vi "lecroy channels to runs.vi"(8 "error in":errorcluster, 9 "Channels in Group":dbl[](array[numeric]), 10 "Crate":i32, 11 "Group Name":string) -> (0 "error out":errorcluster, 2 "Num Channels":i32[](array[numeric]), 3 "First Channel":T1[](array[typedef]) {"Card.Channel" format="%.2f"})   [LabVIEW 2018]
uses:
  archive/CAEN_SY527 v3/CAEN_SY527/subvis/channel.ctl
  <userlib>/_OpenG.lib/array/array.llb/Remove Duplicates from 1D Array (DBL)__ogtk.vi
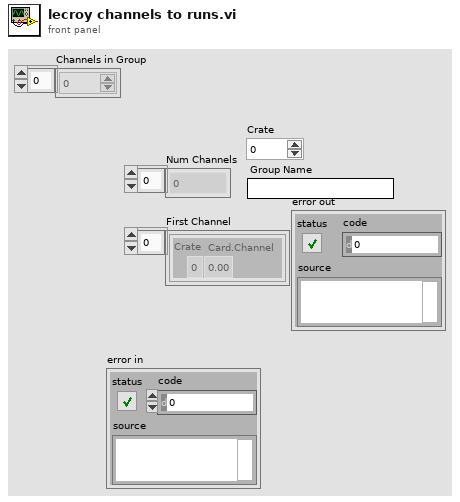
[diagram p1: front panel]
types:
  T1 = typedef "channel.ctl" = cluster{" Card.Channel":dbl, "Crate":i32}
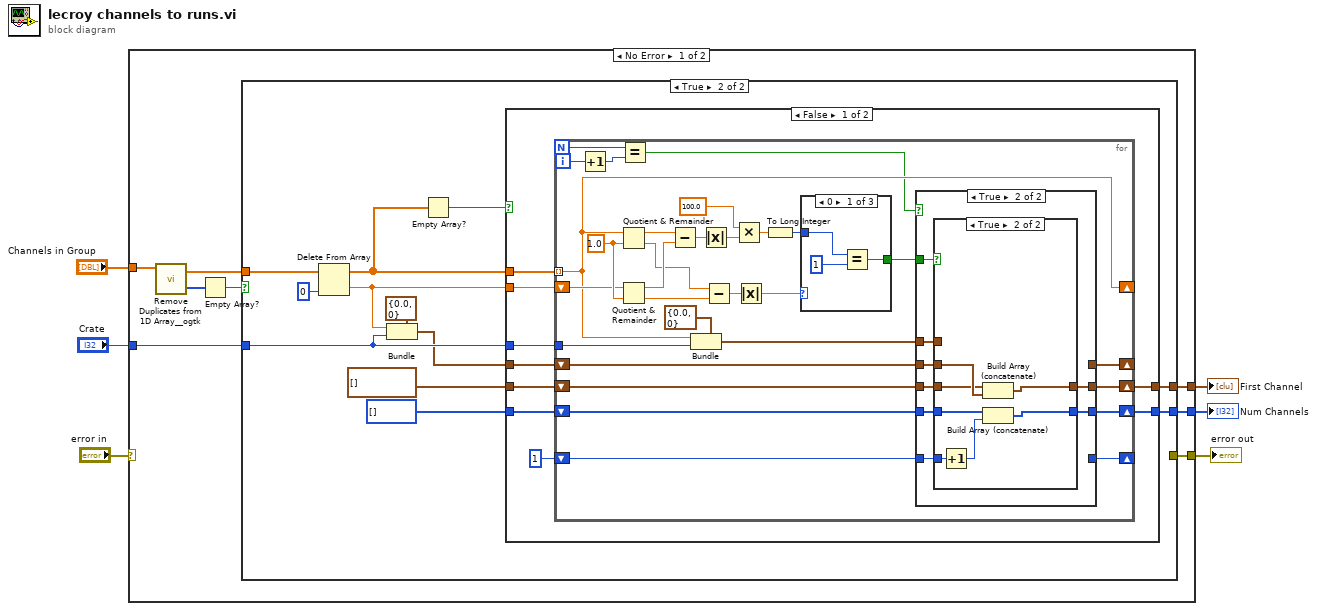
[diagram p0: block diagram]
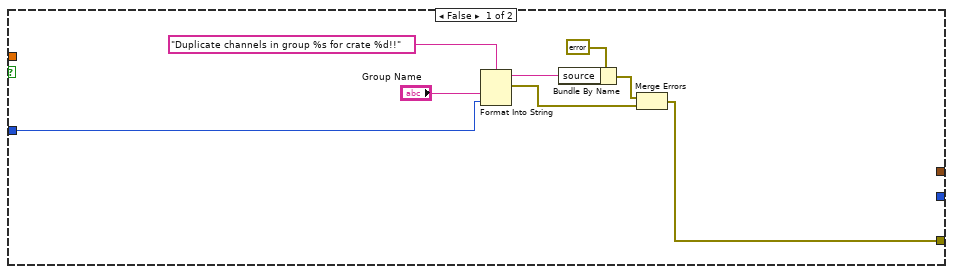
[diagram p2: hidden frame]
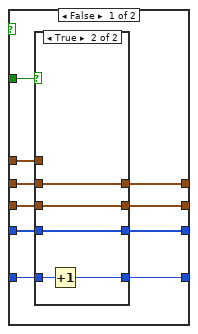
[diagram p3: hidden frame]
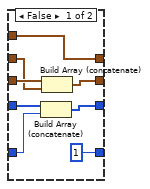
[diagram p4: hidden frame]
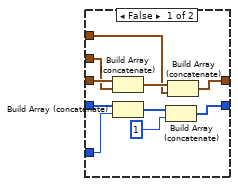
[diagram p5: hidden frame]
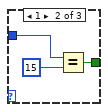
[diagram p6: hidden frame]
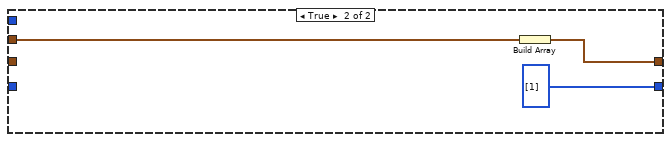
[diagram p8: hidden frame]
diagram:
  n1 = case shown="No Error" "error in" {
    selector: "error in" -> [_ w131]
    tunnel: [w14 _] -> w6
    tunnel: [w13 _] -> w5
    tunnel: "Crate" -> [w12 _]
    tunnel: "Channels in Group" -> [w11 _]
    tunnel: [w7 w131] -> w2
    frame No Error {
      n2 = call-poly <userlib>:"Remove Duplicates from 1D Array__ogtk.vi"("Input Array"=w11) -> ("Output Array"=w10:dbl[], "indices of removed elements"=w9:i32[])
      n3 = Empty Array?(array=w9) -> (empty?=w8:bool)
      n4 = case shown="True" w8 {
        tunnel: [_ w34] -> w14
        tunnel: [_ w33] -> w13
        tunnel: w12 -> [w17 w25]
        tunnel: w10 -> [_ w26]
        tunnel: [w15 _] -> w7
        frame False {
          n5 = Format Into String(format string="Duplicate channels in group %s for crate %d!!" ("source"), "Group Name", w17) -> (resulting string=w20:string, error out=w18:errorcluster)  [unwired: 2 in]
          n6 = Bundle By Name(cluster=errorcluster {"status"=TRUE, "code"=0, "source"=""} ("error constant"), "source"=w20) -> (w19:errorcluster)
          n7 = Merge Errors(w19, w18) -> (w15:errorcluster)
        }
        frame True {
          n8 = Delete From Array(array=w26, index=0) -> (deleted portion=w29:dbl, array with subset deleted=w27:dbl[])  [unwired: 1 in]
          n9 = Bundle(cluster=T1 {" Card.Channel"=0.0, "Crate"=0} ("First Channel"), "Card.Channel"=w29, "Crate"=w25) -> (w24:T1)
          n10 = Empty Array?(array=w27) -> (empty?=w28:bool)
          n11 = case shown="False" w28 {
            tunnel: [w43 i32[] [1]] -> w34
            tunnel: [w42 w128] -> w33
            tunnel: i32[] [] -> [w41 _]
            tunnel: w29 -> [w40 _]
            tunnel: T1[] [] -> [w39 _]
            tunnel: w27 -> [w38 _]
            tunnel: w25 -> [w36 _]
            tunnel: w24 -> [w35 w129]
            frame False {
              n12 = for {
                N -> [w52]
                tunnel: w38 -> [w59] mode=indexing
                shift-right: [w72] -> w42
                shift-left: w39 -> [w65]
                shift-right: [w73] -> w43
                shift-left: w41 -> [w56]
                shift-right: [w59] -> _
                shift-left: w40 -> [w70]
                shift-right: [w64] -> _
                shift-left: 1 ("index") -> [w57]
                tunnel: w36 -> [w60]
                shift-right: [w55] -> _
                shift-left: w35 -> [w54]
                i -> [w51]
                w71 = 1.0 ("y")
                n13 = Increment(x=w51) -> (x+1=w50:i32)
                n14 = Quotient & Remainder(x=w59, y=w71) -> (x-y*floor(x/y)=w69:dbl, floor(x/y)=w66:dbl)
                n15 = Quotient & Remainder(x=w70, y=w71) -> (x-y*floor(x/y)=w68:dbl, floor(x/y)=w67:dbl)
                n16 = Equal?(x=w52, y=w50) -> (x = y?=w49:bool)
                n17 = Subtract(x=w69, y=w68) -> (x-y=w63:dbl)
                n18 = Bundle(cluster=T1 {" Card.Channel"=0.0, "Crate"=0} ("First Channel"), "Card.Channel"=w59, "Crate"=w60) -> (w58:T1)
                n19 = Absolute Value(x=w63) -> (abs(x)=w48:dbl)
                n20 = Subtract(x=w66, y=w67) -> (x-y=w62:dbl)
                n21 = Multiply(x=100.0 ("y"), y=w48) -> (x*y=w45:dbl)
                n22 = Absolute Value(x=w62) -> (abs(x)=w61:dbl)
                n23 = To Long Integer(number=w45) -> (32bit integer=w44:i32)
                n24 = case shown="0" w61 {
                  tunnel: w44 -> [w123 w126 _]
                  tunnel: [w122 w125 _] -> w46
                  frame 0 {
                    n25 = Equal?(x=w123, y=1) -> (x = y?=w122:bool)
                  }
                  frame 1 {
                    n26 = Equal?(x=w126, y=15) -> (x = y?=w125:bool)
                  }
                  frame Default {
                  }
                }
                n27 = case shown="True" w49 {
                  tunnel: [w83 w101] -> w73
                  tunnel: [w82 w104] -> w72
                  tunnel: w46 -> [w81 w99]
                  tunnel: w65 -> [w80 w102]
                  tunnel: [w79 _] -> w64
                  tunnel: w58 -> [w78 w97]
                  tunnel: w57 -> [w77 w100]
                  tunnel: w56 -> [w76 w98]
                  tunnel: [w75 _] -> w55
                  tunnel: w54 -> [w74 w103]
                  frame False {
                    n28 = case shown="True" w81 {
                      tunnel: [w86 w93] -> w83
                      tunnel: [w88 w96] -> w82
                      tunnel: w80 -> [w89 w96]
                      tunnel: [1 w94] -> w79
                      tunnel: w77 -> [w84 w95]
                      tunnel: w78 -> [w90 _]
                      tunnel: w76 -> [w85 w93]
                      tunnel: [w90 w92] -> w75
                      tunnel: w74 -> [w87 w92]
                      frame False {
                        n29 = Build Array (concatenate)(w85, w84) -> (w86:i32[])
                        n30 = Build Array (concatenate)(w89, w87) -> (w88:T1[])
                      }
                      frame True {
                        n31 = Increment(x=w95) -> (x+1=w94:i32)
                      }
                    }
                  }
                  frame True {
                    n32 = case shown="True" w99 {
                      tunnel: [w109 w121] -> w104
                      tunnel: w103 -> [w113 w120]
                      tunnel: w102 -> [w114 w119]
                      tunnel: [w106 w118] -> w101
                      tunnel: w100 -> [w111 w117]
                      tunnel: w98 -> [w112 w115]
                      tunnel: w97 -> [w108 _]
                      frame False {
                        n33 = Build Array (concatenate)(w114, w113) -> (w110:T1[])
                        n34 = Build Array (concatenate)(w112, w111) -> (w107:i32[])
                        n35 = Build Array (concatenate)(w107, 1 ("index")) -> (w106:i32[])
                        n36 = Build Array (concatenate)(w110, w108) -> (w109:T1[])
                      }
                      frame True {
                        n37 = Increment(x=w117) -> (x+1=w116:i32)
                        n38 = Build Array (concatenate)(w119, w120) -> (w121:T1[])
                        n39 = Build Array (concatenate)(w115, w116) -> (w118:i32[])
                      }
                    }
                  }
                }
              }
            }
            frame True {
              n40 = Build Array(w129) -> (w128:T1[])
            }
          }
        }
      }
    }
    frame Error {
    }
  }
  "Num Channels" <- w6
  "First Channel" <- w5
  "error out" <- w2
